vi "Destroy Buffer.vi"(8 "error in (no error)":errorcluster, 11 "Circular Buffer 2D U16 DVR Queue Circular Buffer in":refnum<class "Circular Buffer 2D U16 DVR Queue Circular Buffer.lvclass">) -> (0 "error out":errorcluster, 3 "Circular Buffer 2D U16 DVR Queue Circular Buffer out":refnum<class "Circular Buffer 2D U16 DVR Queue Circular Buffer.lvclass">)   [LabVIEW 2024, in "Circular Buffer 2D U16 DVR Queue Circular Buffer.lvclass"]
uses:
  Circular Buffer 2D U16 DVR Queue Circular Buffer.lvclass
  Circular Buffer 2D U16 DVR Queue Circular Buffer.lvclass/Circular Buffer 2D U16 DVR Queue Circular Buffer.ctl
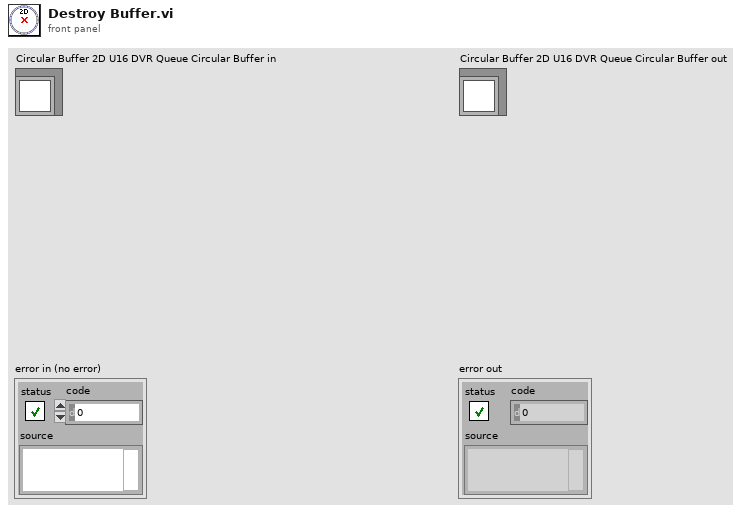
[diagram p1: front panel]
types:
  T1 = typedef "2D U16 DVR Queue.ctl" = refnum<queue>
  T2 = typedef "2D U16 DVR.ctl" = refnum<data-value>
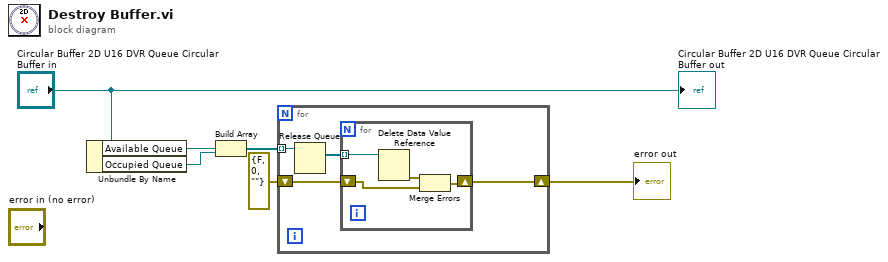
[diagram p0: block diagram]
diagram:
  n1 = Unbundle By Name("Circular Buffer 2D U16 DVR Queue Circular Buffer in") -> ("Available Queue"=w5:T1, "Occupied Queue"=w4:T1)
  n2 = Build Array(w5, w4) -> (w3:T1[])
  n3 = for {
    tunnel: w3 -> [w10] mode=indexing
    shift-right: [w8] -> w1
    shift-left: errorcluster {"status"=FALSE, "code"=0, "source"=""} ("error IO") -> [w7]
    n4 = Release Queue(queue=w10) -> (remaining elements=w9:T2[])  [unwired: 2 in, 2 out]
    n5 = for {
      tunnel: w9 -> [w14] mode=indexing
      shift-right: [w12] -> w8
      shift-left: w7 -> [w11]
      n6 = Delete Data Value Reference(data value reference=w14) -> (error out=w13:errorcluster)  [unwired: 1 in, 1 out]
      n7 = Merge Errors(w13, w11) -> (w12:errorcluster)
    }
  }
  "error out" <- w1
  "Circular Buffer 2D U16 DVR Queue Circular Buffer out" <- "Circular Buffer 2D U16 DVR Queue Circular Buffer in"
